vi "Test - helloDqmhWorldModule - Do Something Else 1.vi"(8 "error in":errorcluster) -> (0 "error out":errorcluster)   [LabVIEW 2023]
doc: "_____\nCreated using DQMH Event Scripter 7.0.0.1280."
uses:
  <vilib>/addons/_JKI Toolkits/Caraya/classes/Assert/Assert Equal Value_Variant.vi
  Libraries/helloDqmhWorldModule/helloDqmhWorldModule.lvlib
  <vilib>/addons/_JKI Toolkits/Caraya/classes/Test/Test.lvclass
  <vilib>/addons/_JKI Toolkits/Caraya/classes/Assert/Assert.lvclass
panel:
  out "Do Something Msg":string
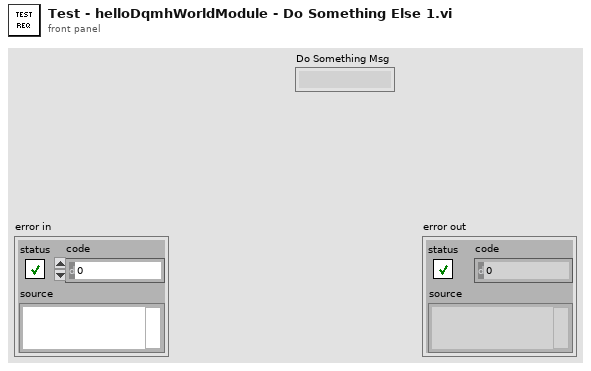
[diagram p1: front panel]
types:
  T1 = typedef "helloDqmhWorldModule.lvlib/Broadcast Events--cluster.ctl" = cluster{"Module Did Init":refnum<user-event>, "Status Updated":refnum<user-event>, "Error Reported":refnum<user-event>, "Did Something":refnum<user-event>, "Module Did Stop":refnum<user-event>, "Update Module Execution Status":refnum<user-event>}
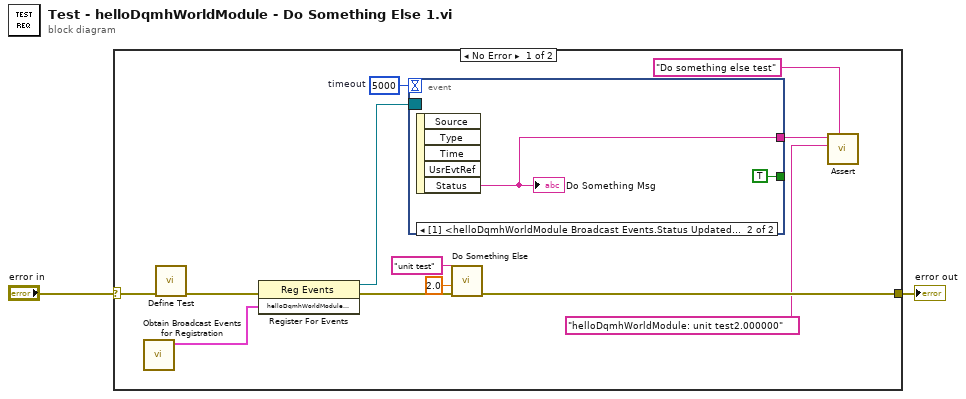
[diagram p0: block diagram]
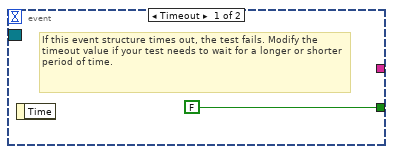
[diagram p2: hidden frame]
diagram:
  n1 = case shown="No Error" "error in" {
    selector: "error in" -> [w6 w18]
    tunnel: [w14 w18] -> w1
    frame No Error {
      w10 = 5000  # timeout
      n2 = call "Obtain Broadcast Events for Registration.vi"() -> ("helloDqmhWorldModule Broadcast Events"=w12:T1)  [unwired: 9 in, 2 out]
      n3 = call <vilib>:"Define Test.vi"("error in (no error)"=w6) -> ("error out"=w5:errorcluster)  [unwired: 9 in, 1 out]
      n4 = register-events(error in=w5, w12) -> (reference out=w11:refnum<event-registration>, error out=w13:errorcluster)  [unwired: 1 in]
      n5 = event shown="[1] <helloDqmhWorldModule Broadcast Events.Status Updated>: User Event" {
        selector: w11 -> [_ _]
        dyn-events: _ -> [_ _]
        timeout: w10 -> [_ _]
        tunnel: [FALSE TRUE] -> _
        tunnel: [_ w16] -> w4
        event Timeout {
          # "If this event structure times out, the test fails. Modify the timeout value if your test needs to wait for a longer or shorter period of time."
          n6 = event-data() -> ()  [unwired: 1 in, 1 out]
        }
        event User Event {
          n7 = event-data() -> ("Status"=w16:string)  [unwired: 1 in, 4 out]
          "Do Something Msg" <- w16
        }
      }
      n8 = call "Do Something Else.vi"("error in"=w13, "X"=2.0, "Do Something Else Message"="unit test") -> ("error out"=w14:errorcluster)  [unwired: 8 in]
      n9 = call-poly <vilib>:"Assert.vi"("Label"="Do something else test" ("Label (VI Title)"), "Y"="helloDqmhWorldModule: unit test2.000000" ("Do Something Msg"), "X"=w4) -> ()  [unwired: 7 in, 2 out]
    }
    frame Error {
    }
  }
  "error out" <- w1
